vi "Launcher.vi"() -> ()   [LabVIEW 2020]
uses:
  UI Actor/UI Actor.lvclass
  C:/Program Files (x86)/National Instruments/LabVIEW 2020/vi.lib/ActorFramework/Actor/Actor.lvclass
  UI Actor/UI Actor.lvclass/UI Actor.ctl
  UI Actor/Write Idioma.vi
  <vilib>/ActorFramework/Actor/Actor.lvclass
panel:
  in  "Idioma":enum16{"Español", "Ingles"}(ring)
  in  "Monedas":enum16{"USD", "MXN"}(ring)
  in  "Productos":enum16{"Cafe", "Coca"}(ring)
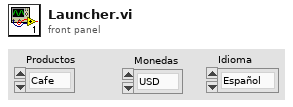
[diagram p1: front panel]
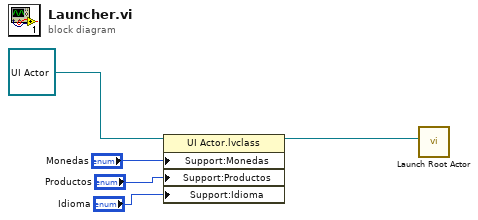
[diagram p0: block diagram]
diagram:
  n1 = property class="UI Actor.lvclass"(reference=refnum<class "UI Actor.lvclass"> refnum ("UI Actor.lvlib:UI Actor.lvclass"), "Support:Monedas"="Monedas", "Support:Productos"="Productos", "Support:Idioma"="Idioma") -> (reference out=w4:refnum<class "UI Actor.lvclass">)  [unwired: 1 in, 1 out]
  n2 = call <vilib>:"Launch Root Actor.vi"("Actor"=w4) -> ()  [unwired: 9 in, 2 out]
